vi "ArrangeRemPan.vi"(8 "error in (no error)":errorcluster caption="entrée d'erreur", 9 "Configuration":i32, 10 "FARefArr":refnum<vi>[](array[refnum]), 11 "PanRef":refnum<vi>) -> (0 "error out":errorcluster caption="sortie d'erreur", 2 "GraphCount":i32, 3 "FARefArrOut":refnum<vi>[](array[refnum]))   [LabVIEW 2019]
uses:
  <vilib>/Utility/miscctls.llb/LVBoundsTypeDef.ctl
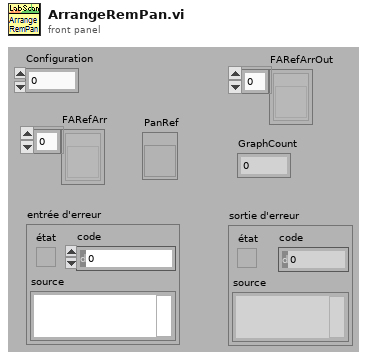
[diagram p1: front panel]
types:
  T1 = typedef "LVBoundsTypeDef.ctl" = cluster{"Width":u32, "Height":u32}
  T2 = typedef "LVPositionTypeDef.ctl" = cluster{"Left":i32, "Top":i32}
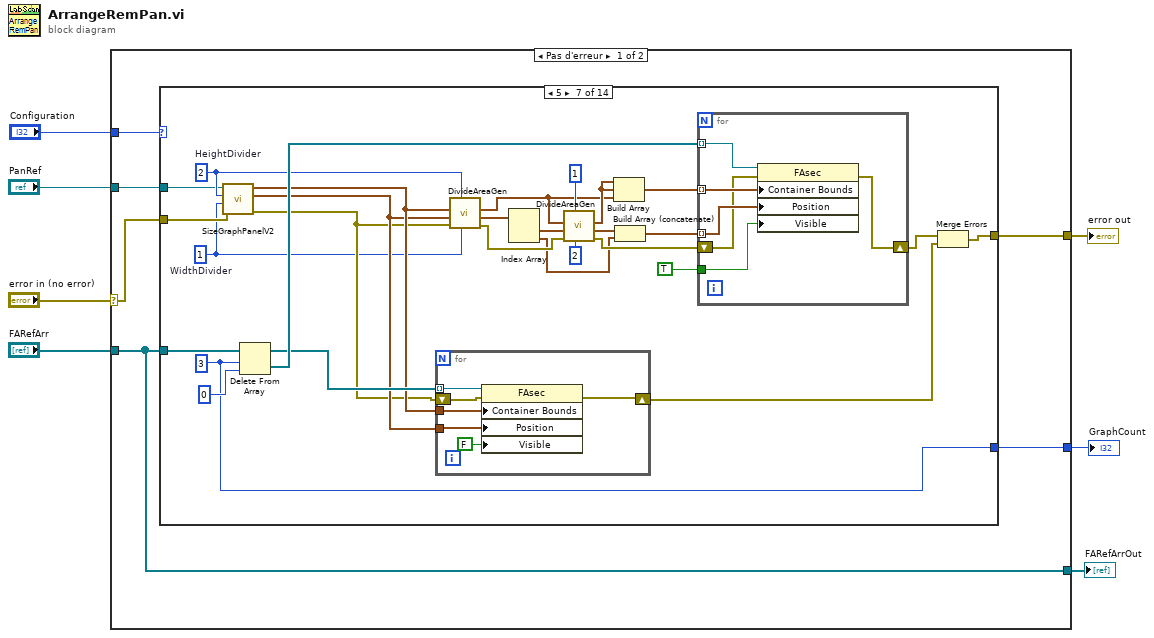
[diagram p0: block diagram]
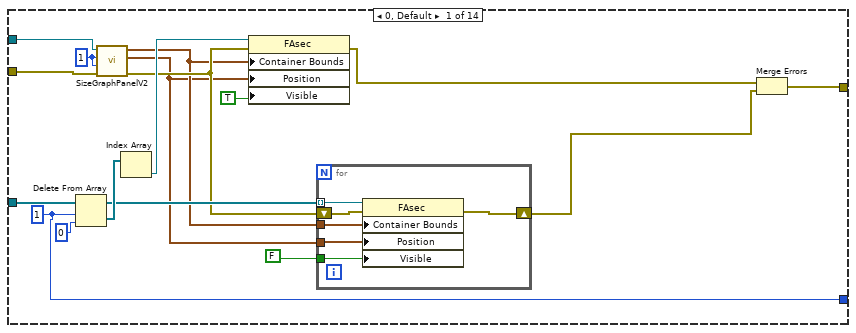
[diagram p2: hidden frame]
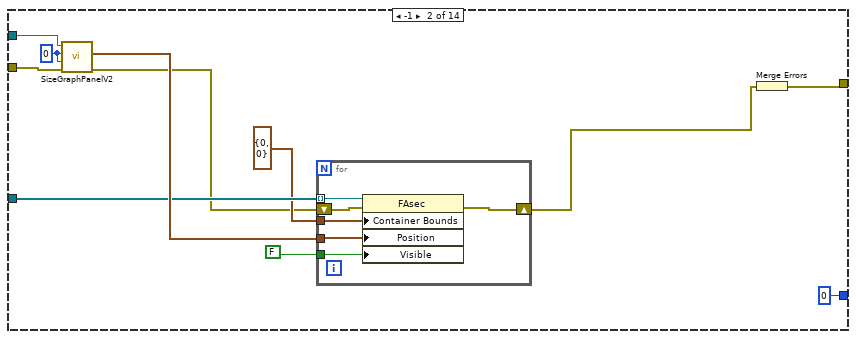
[diagram p3: hidden frame]
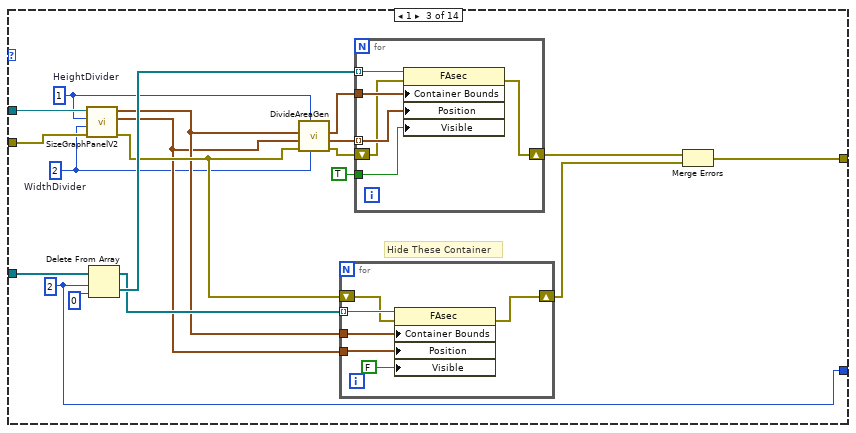
[diagram p4: hidden frame]
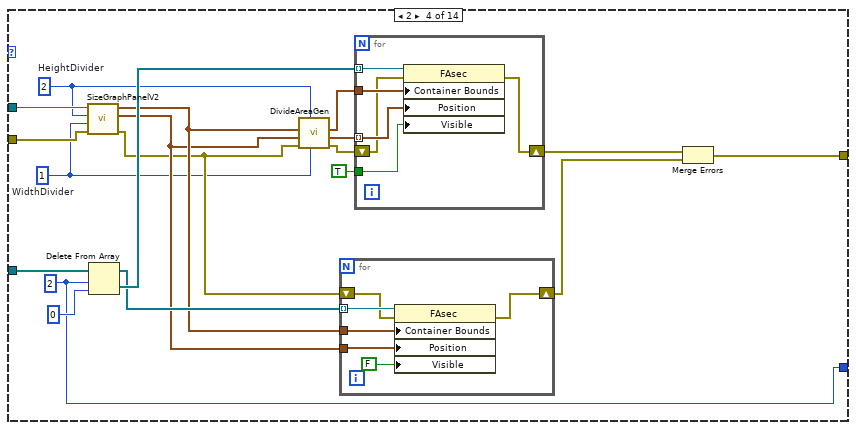
[diagram p5: hidden frame]
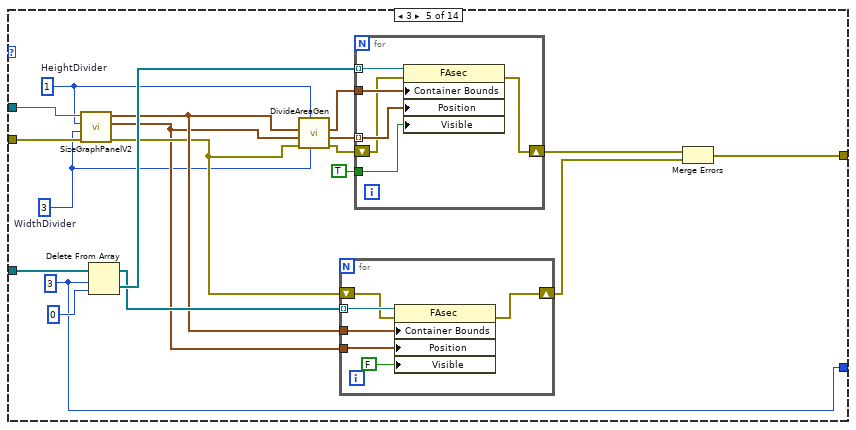
[diagram p6: hidden frame]
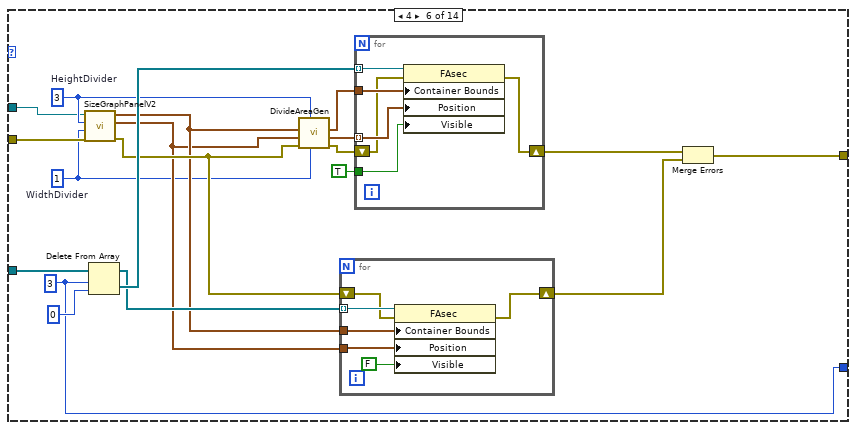
[diagram p7: hidden frame]
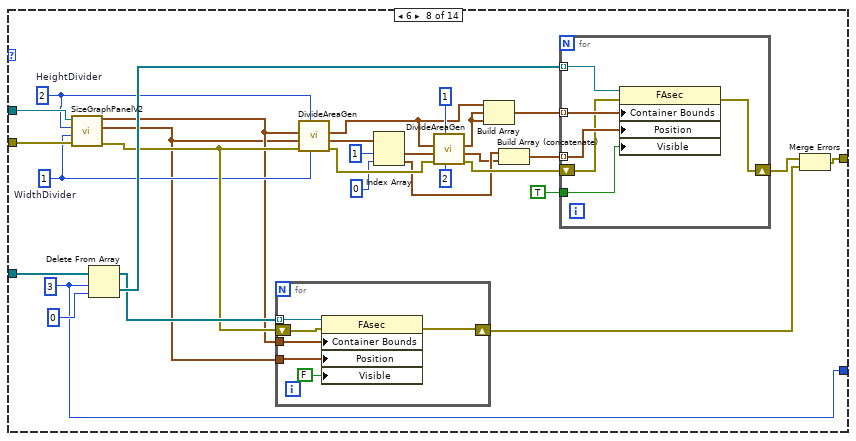
[diagram p8: hidden frame]
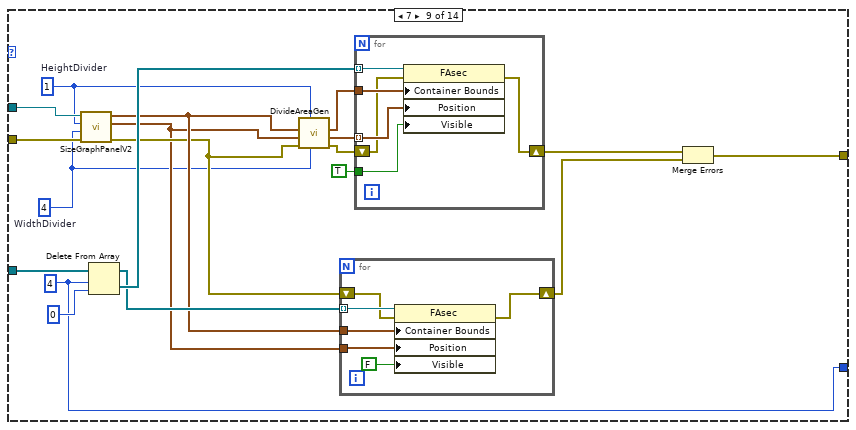
[diagram p9: hidden frame]
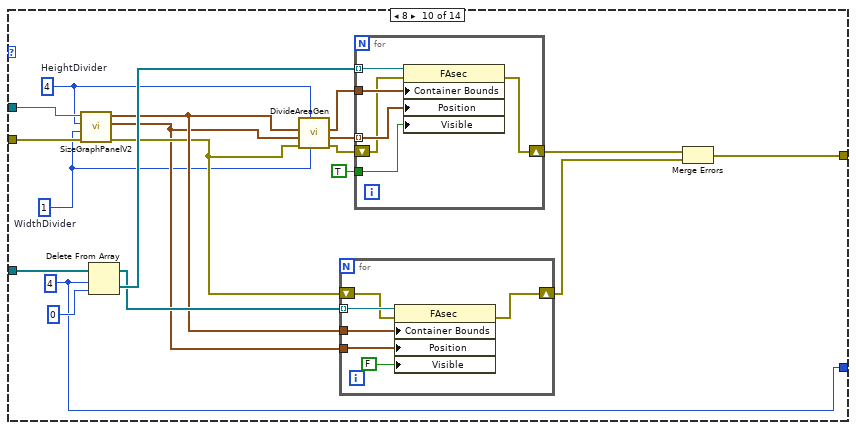
[diagram p10: hidden frame]
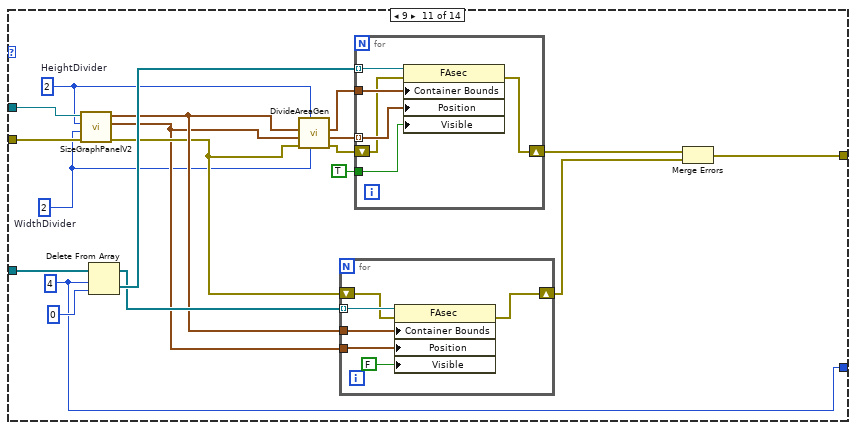
[diagram p11: hidden frame]
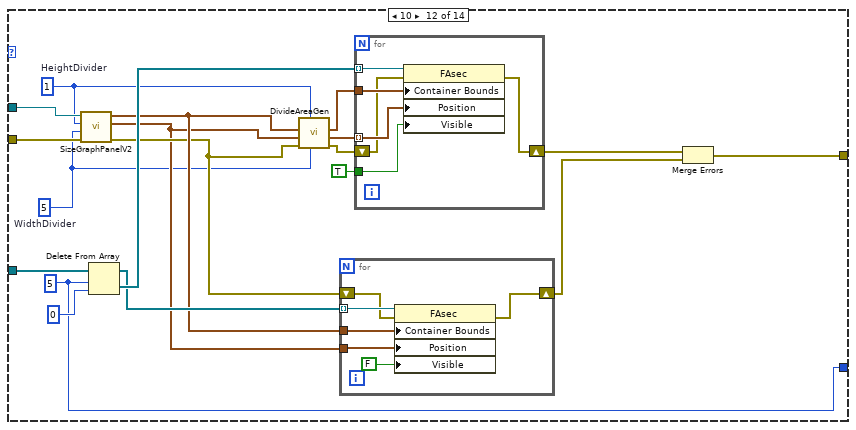
[diagram p12: hidden frame]
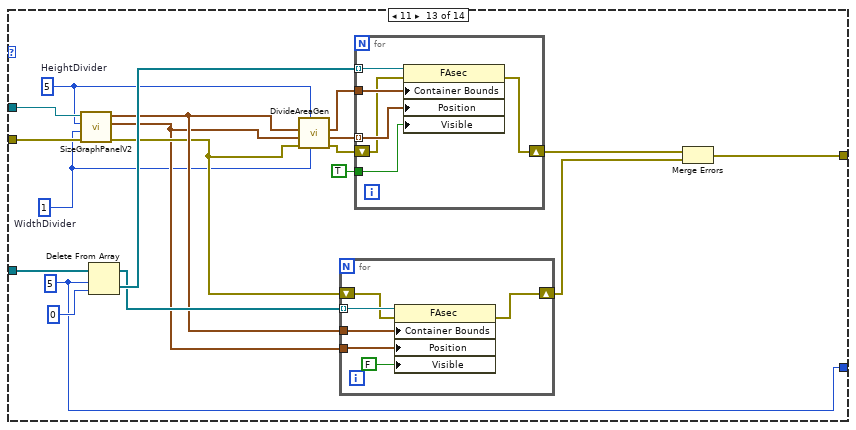
[diagram p13: hidden frame]
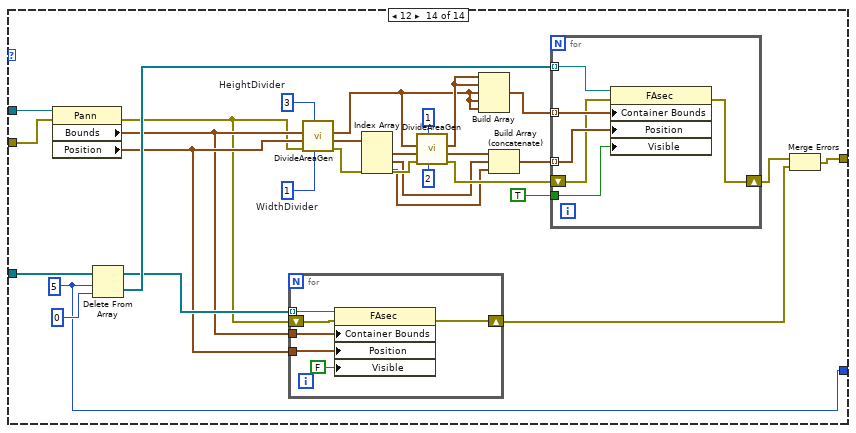
[diagram p14: hidden frame]
diagram:
  n1 = case shown="Pas d'erreur" "error in (no error)" {
    selector: "error in (no error)" -> [w10 w457]
    tunnel: "FARefArr" -> [w8 w456]
    tunnel: "PanRef" -> [w13 _]
    tunnel: "Configuration" -> [w12 _]
    tunnel: [w11 w457] -> w4
    tunnel: [w9 _] -> w2
    tunnel: [w8 w456] -> w1
    frame No Error {
      n2 = case shown="5" w12 {
        tunnel: w13 -> [w18 w38 w56 w90 w122 w148 w178 w222 w266 w297 w328 w359 w390 w443]
        tunnel: w8 -> [w30 w41 w72 w103 w134 w165 w205 w247 w278 w309 w340 w371 w402 w442]
        tunnel: w10 -> [w19 w44 w60 w91 w118 w153 w184 w224 w262 w293 w324 w355 w386 w416]
        tunnel: [w23 w46 w62 w93 w124 w155 w187 w227 w268 w299 w330 w361 w392 w418] -> w11
        tunnel: [w20 0 ("indice") w61 w92 w123 w154 w185 w225 w267 w298 w329 w360 w391 w415] -> w9
        frame 0, Default {
          w17 = 1 ("Height Divider")
          w20 = 1 ("longueur")
          n3 = Delete From Array(array=w30, length=w20, index=0 ("indice")) -> (deleted portion=w28:refnum<vi>[], array with subset deleted=w26:refnum<vi>[])
          n4 = call "SizeGraphPanelV2.vi"("ErrorIn(No Error)"=w19, "Width Divider"=w17, "Height Divider"=w17, "PanRef"=w18) -> ("sortie d'erreur"=w16:errorcluster, "Position"=w14:T2, "cluster de sortie"=w15:T1)  [unwired: 5 in]
          n5 = Index Array(array=w28) -> (element=w27:refnum<vi>)  [unwired: 1 in]
          n6 = property class="FAsec"(reference=w27, error in=w16, "Container Bounds"=w15, "Position"=w14, "Visible"=TRUE) -> (error out=w22:errorcluster)  [unwired: 1 out]
          n7 = for {
            tunnel: w26 -> [w36] mode=indexing
            tunnel: w14 -> [w35]
            tunnel: w15 -> [w34]
            tunnel: FALSE ("Visible") -> [w33]
            shift-right: [w31] -> w21
            shift-left: w16 -> [w32]
            n8 = property class="FAsec"(reference=w36, error in=w32, "Container Bounds"=w34, "Position"=w35, "Visible"=w33) -> (error out=w31:errorcluster)  [unwired: 1 out]
          }
          n9 = Merge Errors(w22, w21) -> (w23:errorcluster)
        }
        frame -1 {
          w43 = 0 ("Height Divider")
          n10 = call "SizeGraphPanelV2.vi"("ErrorIn(No Error)"=w44, "Width Divider"=w43, "Height Divider"=w43, "PanRef"=w38) -> ("sortie d'erreur"=w37:errorcluster, "Position"=w42:T2)  [unwired: 5 in, 1 out]
          n11 = for {
            tunnel: w41 -> [w53] mode=indexing
            tunnel: w42 -> [w52]
            tunnel: T1 {"Width"=0, "Height"=0} ("cluster de sortie") -> [w51]
            tunnel: FALSE ("Visible") -> [w50]
            shift-right: [w48] -> w45
            shift-left: w37 -> [w49]
            n12 = property class="FAsec"(reference=w53, error in=w49, "Container Bounds"=w51, "Position"=w52, "Visible"=w50) -> (error out=w48:errorcluster)  [unwired: 1 out]
          }
          n13 = Merge Errors(w45) -> (w46:errorcluster)
        }
        frame 1 {
          w54 = 2  # WidthDivider
          w55 = 1  # HeightDivider
          w61 = 2 ("indice")
          # "Hide These Container"
          n14 = call "SizeGraphPanelV2.vi"("ErrorIn(No Error)"=w60, "Width Divider"=w54, "Height Divider"=w55, "PanRef"=w56) -> ("sortie d'erreur"=w59:errorcluster, "Position"=w57:T2, "cluster de sortie"=w58:T1)  [unwired: 5 in]
          n15 = Delete From Array(array=w72, length=w61, index=0 ("indice")) -> (deleted portion=w70:refnum<vi>[], array with subset deleted=w66:refnum<vi>[])
          n16 = call <userlib>:"DivideAreaGen.vi"("WidthDivider"=w54, "HeightDivider"=w55, "ErrorIn(No Error)"=w59, "Position"=w57, "Limites"=w58) -> ("sortie d'erreur"=w67:errorcluster, "PositionsOut"=w68:T2[], "LimitsOut"=w69:T1)  [unwired: 4 in]
          n17 = for {
            tunnel: w66 -> [w78] mode=indexing
            tunnel: w57 -> [w77]
            tunnel: w58 -> [w76]
            shift-right: [w73] -> w63
            shift-left: w59 -> [w74]
            n18 = property class="FAsec"(reference=w78, error in=w74, "Container Bounds"=w76, "Position"=w77, "Visible"=FALSE) -> (error out=w73:errorcluster)  [unwired: 1 out]
          }
          n19 = for {
            tunnel: w70 -> [w84] mode=indexing
            tunnel: w69 -> [w83]
            tunnel: w68 -> [w82] mode=indexing
            shift-right: [w80] -> w64
            shift-left: w67 -> [w81]
            tunnel: TRUE ("Visible") -> [w79]
            n20 = property class="FAsec"(reference=w84, error in=w81, "Container Bounds"=w83, "Position"=w82, "Visible"=w79) -> (error out=w80:errorcluster)  [unwired: 1 out]
          }
          n21 = Merge Errors(w64, w63) -> (w62:errorcluster)
        }
        frame 2 {
          w86 = 1  # WidthDivider
          w85 = 2  # HeightDivider
          w92 = 2 ("indice")
          n22 = call "SizeGraphPanelV2.vi"("ErrorIn(No Error)"=w91, "Width Divider"=w86, "Height Divider"=w85, "PanRef"=w90) -> ("sortie d'erreur"=w87:errorcluster, "Position"=w88:T2, "cluster de sortie"=w89:T1)  [unwired: 5 in]
          n23 = Delete From Array(array=w103, length=w92, index=0 ("indice")) -> (deleted portion=w101:refnum<vi>[], array with subset deleted=w97:refnum<vi>[])
          n24 = call <userlib>:"DivideAreaGen.vi"("WidthDivider"=w86, "HeightDivider"=w85, "ErrorIn(No Error)"=w87, "Position"=w88, "Limites"=w89) -> ("sortie d'erreur"=w98:errorcluster, "PositionsOut"=w99:T2[], "LimitsOut"=w100:T1)  [unwired: 4 in]
          n25 = for {
            tunnel: w97 -> [w109] mode=indexing
            tunnel: w88 -> [w108]
            tunnel: w89 -> [w107]
            shift-right: [w104] -> w94
            shift-left: w87 -> [w105]
            n26 = property class="FAsec"(reference=w109, error in=w105, "Container Bounds"=w107, "Position"=w108, "Visible"=FALSE) -> (error out=w104:errorcluster)  [unwired: 1 out]
          }
          n27 = for {
            tunnel: w101 -> [w115] mode=indexing
            tunnel: w100 -> [w114]
            tunnel: w99 -> [w113] mode=indexing
            shift-right: [w111] -> w95
            shift-left: w98 -> [w112]
            tunnel: TRUE ("Visible") -> [w110]
            n28 = property class="FAsec"(reference=w115, error in=w112, "Container Bounds"=w114, "Position"=w113, "Visible"=w110) -> (error out=w111:errorcluster)  [unwired: 1 out]
          }
          n29 = Merge Errors(w95, w94) -> (w93:errorcluster)
        }
        frame 3 {
          w117 = 3  # WidthDivider
          w116 = 1  # HeightDivider
          w123 = 3 ("indice")
          n30 = call "SizeGraphPanelV2.vi"("ErrorIn(No Error)"=w118, "Width Divider"=w117, "Height Divider"=w116, "PanRef"=w122) -> ("sortie d'erreur"=w120:errorcluster, "Position"=w119:T2, "cluster de sortie"=w121:T1)  [unwired: 5 in]
          n31 = Delete From Array(array=w134, length=w123, index=0 ("indice")) -> (deleted portion=w132:refnum<vi>[], array with subset deleted=w128:refnum<vi>[])
          n32 = call <userlib>:"DivideAreaGen.vi"("WidthDivider"=w117, "HeightDivider"=w116, "ErrorIn(No Error)"=w120, "Position"=w119, "Limites"=w121) -> ("sortie d'erreur"=w129:errorcluster, "PositionsOut"=w130:T2[], "LimitsOut"=w131:T1)  [unwired: 4 in]
          n33 = for {
            tunnel: w128 -> [w140] mode=indexing
            tunnel: w119 -> [w139]
            tunnel: w121 -> [w138]
            shift-right: [w135] -> w125
            shift-left: w120 -> [w136]
            n34 = property class="FAsec"(reference=w140, error in=w136, "Container Bounds"=w138, "Position"=w139, "Visible"=FALSE) -> (error out=w135:errorcluster)  [unwired: 1 out]
          }
          n35 = for {
            tunnel: w132 -> [w146] mode=indexing
            tunnel: w131 -> [w145]
            tunnel: w130 -> [w144] mode=indexing
            shift-right: [w142] -> w126
            shift-left: w129 -> [w143]
            tunnel: TRUE ("Visible") -> [w141]
            n36 = property class="FAsec"(reference=w146, error in=w143, "Container Bounds"=w145, "Position"=w144, "Visible"=w141) -> (error out=w142:errorcluster)  [unwired: 1 out]
          }
          n37 = Merge Errors(w126, w125) -> (w124:errorcluster)
        }
        frame 4 {
          w147 = 1  # WidthDivider
          w149 = 3  # HeightDivider
          w154 = 3 ("indice")
          n38 = call "SizeGraphPanelV2.vi"("ErrorIn(No Error)"=w153, "Width Divider"=w147, "Height Divider"=w149, "PanRef"=w148) -> ("sortie d'erreur"=w152:errorcluster, "Position"=w150:T2, "cluster de sortie"=w151:T1)  [unwired: 5 in]
          n39 = Delete From Array(array=w165, length=w154, index=0 ("indice")) -> (deleted portion=w163:refnum<vi>[], array with subset deleted=w159:refnum<vi>[])
          n40 = call <userlib>:"DivideAreaGen.vi"("WidthDivider"=w147, "HeightDivider"=w149, "ErrorIn(No Error)"=w152, "Position"=w150, "Limites"=w151) -> ("sortie d'erreur"=w160:errorcluster, "PositionsOut"=w161:T2[], "LimitsOut"=w162:T1)  [unwired: 4 in]
          n41 = for {
            tunnel: w159 -> [w171] mode=indexing
            tunnel: w150 -> [w170]
            tunnel: w151 -> [w169]
            shift-right: [w166] -> w156
            shift-left: w152 -> [w167]
            n42 = property class="FAsec"(reference=w171, error in=w167, "Container Bounds"=w169, "Position"=w170, "Visible"=FALSE) -> (error out=w166:errorcluster)  [unwired: 1 out]
          }
          n43 = for {
            tunnel: w163 -> [w177] mode=indexing
            tunnel: w162 -> [w176]
            tunnel: w161 -> [w175] mode=indexing
            shift-right: [w173] -> w157
            shift-left: w160 -> [w174]
            tunnel: TRUE ("Visible") -> [w172]
            n44 = property class="FAsec"(reference=w177, error in=w174, "Container Bounds"=w176, "Position"=w175, "Visible"=w172) -> (error out=w173:errorcluster)  [unwired: 1 out]
          }
          n45 = Merge Errors(w157, w156) -> (w155:errorcluster)
        }
        frame 5 {
          w179 = 1  # WidthDivider
          w180 = 2  # HeightDivider
          w185 = 3 ("indice")
          n46 = call "SizeGraphPanelV2.vi"("ErrorIn(No Error)"=w184, "Width Divider"=w179, "Height Divider"=w180, "PanRef"=w178) -> ("sortie d'erreur"=w181:errorcluster, "Position"=w182:T2, "cluster de sortie"=w183:T1)  [unwired: 5 in]
          n47 = Delete From Array(array=w205, length=w185, index=0 ("indice")) -> (deleted portion=w203:refnum<vi>[], array with subset deleted=w189:refnum<vi>[])
          n48 = for {
            tunnel: w189 -> [w211] mode=indexing
            tunnel: w182 -> [w210]
            tunnel: w183 -> [w209]
            shift-right: [w206] -> w186
            shift-left: w181 -> [w207]
            n49 = property class="FAsec"(reference=w211, error in=w207, "Container Bounds"=w209, "Position"=w210, "Visible"=FALSE) -> (error out=w206:errorcluster)  [unwired: 1 out]
          }
          n50 = call <userlib>:"DivideAreaGen.vi"("WidthDivider"=w179, "HeightDivider"=w180, "ErrorIn(No Error)"=w181, "Position"=w182, "Limites"=w183) -> ("sortie d'erreur"=w199:errorcluster, "PositionsOut"=w197:T2[], "LimitsOut"=w193:T1)  [unwired: 4 in]
          n51 = Index Array(array=w197) -> (element #1=w202:T2, element #2=w190:T2)  [unwired: 2 in]
          n52 = call <userlib>:"DivideAreaGen.vi"("WidthDivider"=2, "HeightDivider"=1, "ErrorIn(No Error)"=w199, "Position"=w202, "Limites"=w193) -> ("sortie d'erreur"=w195:errorcluster, "PositionsOut"=w198:T2[], "LimitsOut"=w194:T1)  [unwired: 4 in]
          n53 = Build Array(w194, w194, w193) -> (w192:T1[])
          n54 = Build Array (concatenate)(w198, w190) -> (w196:T2[])
          n55 = for {
            tunnel: w203 -> [w217] mode=indexing
            tunnel: w192 -> [w216] mode=indexing
            tunnel: w196 -> [w215] mode=indexing
            shift-right: [w214] -> w191
            shift-left: w195 -> [w213]
            tunnel: TRUE ("Visible") -> [w212]
            n56 = property class="FAsec"(reference=w217, error in=w213, "Container Bounds"=w216, "Position"=w215, "Visible"=w212) -> (error out=w214:errorcluster)  [unwired: 1 out]
          }
          n57 = Merge Errors(w191, w186) -> (w187:errorcluster)
        }
        frame 6 {
          w220 = 1  # WidthDivider
          w221 = 2  # HeightDivider
          w225 = 3 ("indice")
          n58 = call "SizeGraphPanelV2.vi"("ErrorIn(No Error)"=w224, "Width Divider"=w220, "Height Divider"=w221, "PanRef"=w222) -> ("sortie d'erreur"=w223:errorcluster, "Position"=w218:T2, "cluster de sortie"=w219:T1)  [unwired: 5 in]
          n59 = Delete From Array(array=w247, length=w225, index=0 ("indice")) -> (deleted portion=w245:refnum<vi>[], array with subset deleted=w228:refnum<vi>[])
          n60 = for {
            tunnel: w228 -> [w253] mode=indexing
            tunnel: w218 -> [w252]
            tunnel: w219 -> [w251]
            shift-right: [w248] -> w226
            shift-left: w223 -> [w249]
            n61 = property class="FAsec"(reference=w253, error in=w249, "Container Bounds"=w251, "Position"=w252, "Visible"=FALSE) -> (error out=w248:errorcluster)  [unwired: 1 out]
          }
          n62 = call <userlib>:"DivideAreaGen.vi"("WidthDivider"=w220, "HeightDivider"=w221, "ErrorIn(No Error)"=w223, "Position"=w218, "Limites"=w219) -> ("sortie d'erreur"=w242:errorcluster, "PositionsOut"=w241:T2[], "LimitsOut"=w234:T1)  [unwired: 4 in]
          n63 = Index Array(array=w241, index #1=1 ("indice"), index #2=0 ("indice")) -> (element #1=w232:T2, element #2=w231:T2)
          n64 = call <userlib>:"DivideAreaGen.vi"("WidthDivider"=2, "HeightDivider"=1, "ErrorIn(No Error)"=w242, "Position"=w232, "Limites"=w234) -> ("sortie d'erreur"=w239:errorcluster, "PositionsOut"=w230:T2[], "LimitsOut"=w233:T1)  [unwired: 4 in]
          n65 = Build Array(w234, w233, w233) -> (w238:T1[])
          n66 = Build Array (concatenate)(w231, w230) -> (w240:T2[])
          n67 = for {
            tunnel: w245 -> [w259] mode=indexing
            tunnel: w238 -> [w258] mode=indexing
            tunnel: w240 -> [w257] mode=indexing
            shift-right: [w256] -> w237
            shift-left: w239 -> [w255]
            tunnel: TRUE ("Visible") -> [w254]
            n68 = property class="FAsec"(reference=w259, error in=w255, "Container Bounds"=w258, "Position"=w257, "Visible"=w254) -> (error out=w256:errorcluster)  [unwired: 1 out]
          }
          n69 = Merge Errors(w237, w226) -> (w227:errorcluster)
        }
        frame 7 {
          w261 = 4  # WidthDivider
          w260 = 1  # HeightDivider
          w267 = 4 ("indice")
          n70 = call "SizeGraphPanelV2.vi"("ErrorIn(No Error)"=w262, "Width Divider"=w261, "Height Divider"=w260, "PanRef"=w266) -> ("sortie d'erreur"=w264:errorcluster, "Position"=w263:T2, "cluster de sortie"=w265:T1)  [unwired: 5 in]
          n71 = Delete From Array(array=w278, length=w267, index=0 ("indice")) -> (deleted portion=w276:refnum<vi>[], array with subset deleted=w272:refnum<vi>[])
          n72 = call <userlib>:"DivideAreaGen.vi"("WidthDivider"=w261, "HeightDivider"=w260, "ErrorIn(No Error)"=w264, "Position"=w263, "Limites"=w265) -> ("sortie d'erreur"=w273:errorcluster, "PositionsOut"=w274:T2[], "LimitsOut"=w275:T1)  [unwired: 4 in]
          n73 = for {
            tunnel: w272 -> [w284] mode=indexing
            tunnel: w263 -> [w283]
            tunnel: w265 -> [w282]
            shift-right: [w279] -> w269
            shift-left: w264 -> [w280]
            n74 = property class="FAsec"(reference=w284, error in=w280, "Container Bounds"=w282, "Position"=w283, "Visible"=FALSE) -> (error out=w279:errorcluster)  [unwired: 1 out]
          }
          n75 = for {
            tunnel: w276 -> [w290] mode=indexing
            tunnel: w275 -> [w289]
            tunnel: w274 -> [w288] mode=indexing
            shift-right: [w286] -> w270
            shift-left: w273 -> [w287]
            tunnel: TRUE ("Visible") -> [w285]
            n76 = property class="FAsec"(reference=w290, error in=w287, "Container Bounds"=w289, "Position"=w288, "Visible"=w285) -> (error out=w286:errorcluster)  [unwired: 1 out]
          }
          n77 = Merge Errors(w270, w269) -> (w268:errorcluster)
        }
        frame 8 {
          w292 = 1  # WidthDivider
          w291 = 4  # HeightDivider
          w298 = 4 ("indice")
          n78 = call "SizeGraphPanelV2.vi"("ErrorIn(No Error)"=w293, "Width Divider"=w292, "Height Divider"=w291, "PanRef"=w297) -> ("sortie d'erreur"=w295:errorcluster, "Position"=w294:T2, "cluster de sortie"=w296:T1)  [unwired: 5 in]
          n79 = Delete From Array(array=w309, length=w298, index=0 ("indice")) -> (deleted portion=w307:refnum<vi>[], array with subset deleted=w303:refnum<vi>[])
          n80 = call <userlib>:"DivideAreaGen.vi"("WidthDivider"=w292, "HeightDivider"=w291, "ErrorIn(No Error)"=w295, "Position"=w294, "Limites"=w296) -> ("sortie d'erreur"=w304:errorcluster, "PositionsOut"=w305:T2[], "LimitsOut"=w306:T1)  [unwired: 4 in]
          n81 = for {
            tunnel: w303 -> [w315] mode=indexing
            tunnel: w294 -> [w314]
            tunnel: w296 -> [w313]
            shift-right: [w310] -> w300
            shift-left: w295 -> [w311]
            n82 = property class="FAsec"(reference=w315, error in=w311, "Container Bounds"=w313, "Position"=w314, "Visible"=FALSE) -> (error out=w310:errorcluster)  [unwired: 1 out]
          }
          n83 = for {
            tunnel: w307 -> [w321] mode=indexing
            tunnel: w306 -> [w320]
            tunnel: w305 -> [w319] mode=indexing
            shift-right: [w317] -> w301
            shift-left: w304 -> [w318]
            tunnel: TRUE ("Visible") -> [w316]
            n84 = property class="FAsec"(reference=w321, error in=w318, "Container Bounds"=w320, "Position"=w319, "Visible"=w316) -> (error out=w317:errorcluster)  [unwired: 1 out]
          }
          n85 = Merge Errors(w301, w300) -> (w299:errorcluster)
        }
        frame 9 {
          w323 = 2  # WidthDivider
          w322 = 2  # HeightDivider
          w329 = 4 ("indice")
          n86 = call "SizeGraphPanelV2.vi"("ErrorIn(No Error)"=w324, "Width Divider"=w323, "Height Divider"=w322, "PanRef"=w328) -> ("sortie d'erreur"=w326:errorcluster, "Position"=w325:T2, "cluster de sortie"=w327:T1)  [unwired: 5 in]
          n87 = Delete From Array(array=w340, length=w329, index=0 ("indice")) -> (deleted portion=w338:refnum<vi>[], array with subset deleted=w334:refnum<vi>[])
          n88 = call <userlib>:"DivideAreaGen.vi"("WidthDivider"=w323, "HeightDivider"=w322, "ErrorIn(No Error)"=w326, "Position"=w325, "Limites"=w327) -> ("sortie d'erreur"=w335:errorcluster, "PositionsOut"=w336:T2[], "LimitsOut"=w337:T1)  [unwired: 4 in]
          n89 = for {
            tunnel: w334 -> [w346] mode=indexing
            tunnel: w325 -> [w345]
            tunnel: w327 -> [w344]
            shift-right: [w341] -> w331
            shift-left: w326 -> [w342]
            n90 = property class="FAsec"(reference=w346, error in=w342, "Container Bounds"=w344, "Position"=w345, "Visible"=FALSE) -> (error out=w341:errorcluster)  [unwired: 1 out]
          }
          n91 = for {
            tunnel: w338 -> [w352] mode=indexing
            tunnel: w337 -> [w351]
            tunnel: w336 -> [w350] mode=indexing
            shift-right: [w348] -> w332
            shift-left: w335 -> [w349]
            tunnel: TRUE ("Visible") -> [w347]
            n92 = property class="FAsec"(reference=w352, error in=w349, "Container Bounds"=w351, "Position"=w350, "Visible"=w347) -> (error out=w348:errorcluster)  [unwired: 1 out]
          }
          n93 = Merge Errors(w332, w331) -> (w330:errorcluster)
        }
        frame 10 {
          w354 = 5  # WidthDivider
          w353 = 1  # HeightDivider
          w360 = 5 ("indice")
          n94 = call "SizeGraphPanelV2.vi"("ErrorIn(No Error)"=w355, "Width Divider"=w354, "Height Divider"=w353, "PanRef"=w359) -> ("sortie d'erreur"=w357:errorcluster, "Position"=w356:T2, "cluster de sortie"=w358:T1)  [unwired: 5 in]
          n95 = Delete From Array(array=w371, length=w360, index=0 ("indice")) -> (deleted portion=w369:refnum<vi>[], array with subset deleted=w365:refnum<vi>[])
          n96 = call <userlib>:"DivideAreaGen.vi"("WidthDivider"=w354, "HeightDivider"=w353, "ErrorIn(No Error)"=w357, "Position"=w356, "Limites"=w358) -> ("sortie d'erreur"=w366:errorcluster, "PositionsOut"=w367:T2[], "LimitsOut"=w368:T1)  [unwired: 4 in]
          n97 = for {
            tunnel: w365 -> [w377] mode=indexing
            tunnel: w356 -> [w376]
            tunnel: w358 -> [w375]
            shift-right: [w372] -> w362
            shift-left: w357 -> [w373]
            n98 = property class="FAsec"(reference=w377, error in=w373, "Container Bounds"=w375, "Position"=w376, "Visible"=FALSE) -> (error out=w372:errorcluster)  [unwired: 1 out]
          }
          n99 = for {
            tunnel: w369 -> [w383] mode=indexing
            tunnel: w368 -> [w382]
            tunnel: w367 -> [w381] mode=indexing
            shift-right: [w379] -> w363
            shift-left: w366 -> [w380]
            tunnel: TRUE ("Visible") -> [w378]
            n100 = property class="FAsec"(reference=w383, error in=w380, "Container Bounds"=w382, "Position"=w381, "Visible"=w378) -> (error out=w379:errorcluster)  [unwired: 1 out]
          }
          n101 = Merge Errors(w363, w362) -> (w361:errorcluster)
        }
        frame 11 {
          w385 = 1  # WidthDivider
          w384 = 5  # HeightDivider
          w391 = 5 ("indice")
          n102 = call "SizeGraphPanelV2.vi"("ErrorIn(No Error)"=w386, "Width Divider"=w385, "Height Divider"=w384, "PanRef"=w390) -> ("sortie d'erreur"=w388:errorcluster, "Position"=w387:T2, "cluster de sortie"=w389:T1)  [unwired: 5 in]
          n103 = Delete From Array(array=w402, length=w391, index=0 ("indice")) -> (deleted portion=w400:refnum<vi>[], array with subset deleted=w396:refnum<vi>[])
          n104 = call <userlib>:"DivideAreaGen.vi"("WidthDivider"=w385, "HeightDivider"=w384, "ErrorIn(No Error)"=w388, "Position"=w387, "Limites"=w389) -> ("sortie d'erreur"=w397:errorcluster, "PositionsOut"=w398:T2[], "LimitsOut"=w399:T1)  [unwired: 4 in]
          n105 = for {
            tunnel: w396 -> [w408] mode=indexing
            tunnel: w387 -> [w407]
            tunnel: w389 -> [w406]
            shift-right: [w403] -> w393
            shift-left: w388 -> [w404]
            n106 = property class="FAsec"(reference=w408, error in=w404, "Container Bounds"=w406, "Position"=w407, "Visible"=FALSE) -> (error out=w403:errorcluster)  [unwired: 1 out]
          }
          n107 = for {
            tunnel: w400 -> [w414] mode=indexing
            tunnel: w399 -> [w413]
            tunnel: w398 -> [w412] mode=indexing
            shift-right: [w410] -> w394
            shift-left: w397 -> [w411]
            tunnel: TRUE ("Visible") -> [w409]
            n108 = property class="FAsec"(reference=w414, error in=w411, "Container Bounds"=w413, "Position"=w412, "Visible"=w409) -> (error out=w410:errorcluster)  [unwired: 1 out]
          }
          n109 = Merge Errors(w394, w393) -> (w392:errorcluster)
        }
        frame 12 {
          w438 = 1  # WidthDivider
          w439 = 3  # HeightDivider
          w415 = 5 ("indice")
          n110 = property class="Pann"(reference=w443, error in=w416) -> (error out=w419:errorcluster, "Bounds"=w423:T1, "Position"=w424:T2)  [unwired: 1 out]
          n111 = Delete From Array(array=w442, length=w415, index=0 ("indice")) -> (deleted portion=w440:refnum<vi>[], array with subset deleted=w425:refnum<vi>[])
          n112 = for {
            tunnel: w425 -> [w449] mode=indexing
            tunnel: w424 -> [w448]
            tunnel: w423 -> [w447]
            shift-right: [w444] -> w417
            shift-left: w419 -> [w445]
            n113 = property class="FAsec"(reference=w449, error in=w445, "Container Bounds"=w447, "Position"=w448, "Visible"=FALSE) -> (error out=w444:errorcluster)  [unwired: 1 out]
          }
          n114 = call <userlib>:"DivideAreaGen.vi"("WidthDivider"=w438, "HeightDivider"=w439, "ErrorIn(No Error)"=w419, "Position"=w424, "Limites"=w423) -> ("sortie d'erreur"=w434:errorcluster, "PositionsOut"=w432:T2[], "LimitsOut"=w421:T1)  [unwired: 4 in]
          n115 = Index Array(array=w432) -> (element #1=w437:T2, element #2=w426:T2, element #3=w420:T2)  [unwired: 3 in]
          n116 = call <userlib>:"DivideAreaGen.vi"("WidthDivider"=2, "HeightDivider"=1, "ErrorIn(No Error)"=w434, "Position"=w437, "Limites"=w421) -> ("sortie d'erreur"=w430:errorcluster, "PositionsOut"=w433:T2[], "LimitsOut"=w429:T1)  [unwired: 4 in]
          n117 = Build Array(w429, w429, w421, w421, w421) -> (w428:T1[])
          n118 = Build Array (concatenate)(w433, w426, w420) -> (w431:T2[])
          n119 = for {
            tunnel: w440 -> [w455] mode=indexing
            tunnel: w428 -> [w454] mode=indexing
            tunnel: w431 -> [w453] mode=indexing
            shift-right: [w452] -> w427
            shift-left: w430 -> [w451]
            tunnel: TRUE ("Visible") -> [w450]
            n120 = property class="FAsec"(reference=w455, error in=w451, "Container Bounds"=w454, "Position"=w453, "Visible"=w450) -> (error out=w452:errorcluster)  [unwired: 1 out]
          }
          n121 = Merge Errors(w427, w417) -> (w418:errorcluster)
        }
      }
    }
    frame Error {
    }
  }
  "error out" <- w4
  "GraphCount" <- w2
  "FARefArrOut" <- w1
